vi "Authorization Get Feature.vi"(8 "error in (no error)":errorcluster, 11 "Feature Name":string) -> (0 "error out":errorcluster, 2 "Authorized?":bool, 3 "Feature Name Out":string)   [LabVIEW 2011]
doc: "GetAuthorization() gets the level at which the protected program is authorized to run along with the options enabled or an authorization failure code. It is also used to decrement the number of runs, if the application is restricted by runs.\n\nGetAuthorization() can be called at your discretion to determine the level of authorization that the user is granted. It can also be called to decrement the number of uses the program has left if it is restricted by number of runs. Call this function after calling any function that changes the license state, such as SaveSiteKey(), TransferOut() or TransferIn(), so that the program can alter its behavior according to the change that has occurred.\n\nValue Meaning\n>0 The program is authorized to run. The program has a floating license and more users are requesting to use the program than the license allows. The number indicates how many users must quit before the next user is authorized to run. CrypKey queues requests for access and provides access on a first-come, first-served basis.\n0 The program is authorized to run.\n-1 CrypKey has not been initialized.\n-2 An attempt is being made to run the protected program from a floppy disk.\n-3 Could not read the site key file.\n-4 The program has never been authorized at the current site.\n-5 The program is moved or the password is incorrect.\n-6 The Master Key is not correct for this program.\n-7 The site key file is damaged or tampered with.\n-8 The system time is set to a date earlier than the date on which the Site Key was issued.\n-9 The program is restricted by days and the system time is set back.\n-10 The program is restricted by days and the time has expired.\n-11 The program is restricted by runs and the number allowed is reached.\n-12 The user tried to perform an operation that requires more runs than are available.\n-13 The restriction file is deleted.\n-14 The restriction file is damaged or tampered with.\n-15 The restriction file is moved or overwritten.\n-16 The user has attempted to reuse an old site key.\n-17 Could not open or read the network user table file.\n-18 More people are using the protected program than SLAPI can handle.\n-19 An attempt is being made to run the program in client/server mode and a floating license has not been issued for the site.\n-20 .RST file is write protected \n-21 Computer clock tampering detected \n-22 Application site key is moved or copied \n\nThe options are single bits of information that can be turned on or off individually when a license is created using the Site Key Generator. The options exist so that you can turn on or off different features of your product. The options are stored in a numerical sequence starting at one with the high-end bit of the oplevel 32-bit value. The remaining bits are used to hold the level number.\nThe level is a number that is set by the Site Key Generator. It incrementally controls the quality of some services your software provides, such as the number of records allowed for a database. The maximum level depends on the number of options you have configured.\nThere are 32 bits available to both the option and level values."
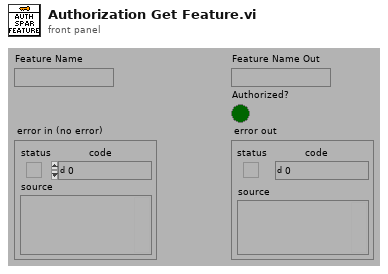
[diagram p1: front panel]
types:
  T1 = enum32{"invalid app kind", "Development System", "Run Time System", "Student Edition", "Embedded LabVIEW", "Evaluation", "Custom"}
  T2 = typedef "Authorization Data.ctl" = cluster{"Valid":bool, "Seats":i32, "Expire Time":timestamp, "Last Access Time":timestamp, "Product ID":string, "Hardware ID":string, "Spartan Serial Number":string, "Feature":cluster{"#attributes":cluster{"Name":string, "Value":string}}[]}
  T3 = cluster{"#attributes":cluster{"Name":string, "Value":string}}[]
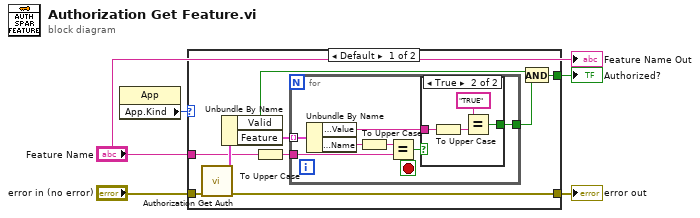
[diagram p0: block diagram]
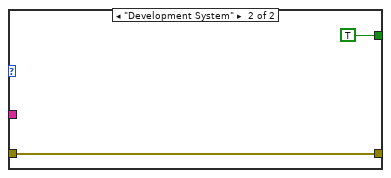
[diagram p3: hidden frame]
diagram:
  n1 = property class="App"() -> ("App.Kind"=w1:T1)  [unwired: 2 in, 2 out]
  n2 = case shown="Default" w1 {
    tunnel: "error in (no error)" -> [w14 w27]
    tunnel: [w13 w27] -> w4
    tunnel: [w7 TRUE] -> w3
    tunnel: "Feature Name" -> [w6 _]
    frame Default {
      n3 = call "Authorization Get Auth.vi"("error in (no error)"=w14) -> ("error out"=w13:errorcluster, "Authorization"=w12:T2)  [unwired: 9 in]
      n4 = Unbundle By Name(w12) -> ("Valid"=w9:bool, "Feature"=w11:T3)
      n5 = To Upper Case(1:w6) -> (0:w10:string)
      n6 = for {
        tunnel: w11 -> [w21] mode=indexing
        tunnel: w10 -> [w18]
        tunnel: [w15] -> w8
        stop <- w17 stop-if-true
        n7 = Unbundle By Name(w21) -> ("#attributes.Value"=w16:string, "#attributes.Name"=w20:string)
        n8 = To Upper Case(1:w20) -> (0:w19:string)
        n9 = Equal?(x=w19, y=w18) -> (x = y?=w17:bool)
        n10 = case shown="True" w17 {
          tunnel: w16 -> [_ w25]
          tunnel: [_ w22] -> w15
          frame False {
          }
          frame True {
            n11 = To Upper Case(1:w25) -> (0:w24:string)
            n12 = Equal?(x="TRUE", y=w24) -> (x = y?=w22:bool)
          }
        }
      }
      n13 = And(x=w9, y=w8) -> (x .and. y?=w7:bool)
    }
    frame "Development System" {
    }
  }
  "error out" <- w4
  "Authorized?" <- w3
  "Feature Name Out" <- "Feature Name"
